vi "PH_BackreflectionMeas.get relevant Data.vi"(0 "i ref in":refnum<vi>, 5 "error in":errorcluster) -> (14 "i ref out":refnum<vi>, 16 "low Energy Waveform":waveform(dbl), 17 "high Energy Waveform":waveform(dbl), 19 "error out":errorcluster)   [LabVIEW 2014, in "PH_BackreflectionMeas.lvlib"]
doc: "This VI gets - depending on the Alignment or shot Mode - the relevant data."
uses:
  PH_BackreflectionMeas.lvlib
  PH_Devices/PH_TKTDS-30xx/PH_TKTDS-30xx.lvlib
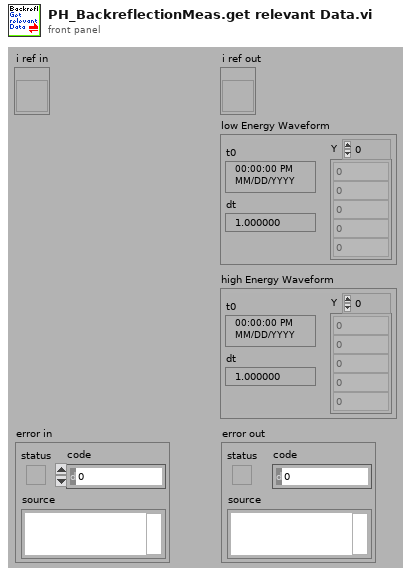
[diagram p1: front panel]
types:
  T1 = typedef "PH_TKTDS-30xx.lvlib/PH_TKTDS-30xx.i attribute.ctl" = cluster{"Default VISA Resource":string, "VISA Resource Name":refnum<visa-resource-name>, "Revision":cluster{"Instrument Driver":string, "Instrument Firmware":string}, "Selftest":cluster{"Result":u32, "Message":string}, "Channels":T2[], "Trigger Configuration":T4, "Acquisition Configuration":T5, "Fetched Waveforms":T6[], "GUI Refs":T7, "State":T8, "Error Message":string, "Allow Prdc Loop?":bool}
  T2 = typedef "PH_TKTDS-30xx.lvlib/PH_TKTDS-30xx.Channel Config.ctl" = cluster{"Channel Name":string, "Input Impedance":string, "Max Input Frequency":string, "Vertical Coupling":i32, "Channel Enabled":bool, "Probe Attenuation":dbl, "Vertical Range":dbl, "Vertical Offset":dbl, "Waveform Limits":T3}
  T3 = typedef "PH_TKTDS-30xx.lvlib/PH_TKTDS-30xx.Waveform Limits.ctl" = cluster{"Start":i32, "End":i32}
  T4 = typedef "PH_TKTDS-30xx.lvlib/PH_TKTDS-30xx.Trigger Config.ctl" = cluster{"Source":string, "Slope":i32, "Level [V]":dbl}
  T5 = typedef "PH_TKTDS-30xx.lvlib/PH_TKTDS-30xx.Acquisition Config.ctl" = cluster{"Time base":dbl, "Record Length":u16, "Start Time":dbl, "Type":i32, "Continuous":bool}
  T6 = typedef "PH_TKTDS-30xx.lvlib/PH_TKTDS-30xx.fetched Waveform.ctl" = cluster{"Source":string, "Actual Points":u32, "Initial X":dbl, "X Increment":dbl, "Waveform Array":dbl[]}
  T7 = typedef "PH_TKTDS-30xx.lvlib/PH_TKTDS-30xx.GUI Refs.ctl" = cluster{"Trigger":refnum<vi>, "Acquisition":refnum<vi>, "State":refnum<vi>, "Delete":refnum<vi>, "Channel to be positioned":refnum<vi>, "Postion":refnum<vi>, "Display Intensity":refnum<vi>, "VISA Resource":refnum<vi>, "Channels":refnum<vi>[], "Graphs":refnum<vi>[]}
  T8 = typedef "PH_StatusHandler.lvlib/PH_StatusHandler.Status.ctl" = i16
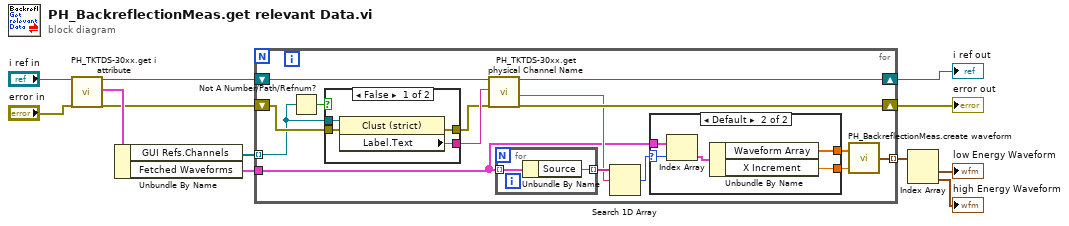
[diagram p0: block diagram]
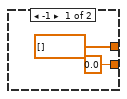
[diagram p2: hidden frame]
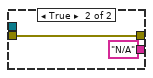
[diagram p3: hidden frame]
diagram:
  n1 = call "PH_TKTDS-30xx.get i attribute.vi"("i ref in"="i ref in", "error in (no error)"="error in") -> ("i ref out"=w7:refnum<vi>, "i attribute"=w12:T1, "error out"=w10:errorcluster)  [unwired: 15 in]
  n2 = Unbundle By Name(w12) -> ("GUI Refs.Channels"=w11:refnum<vi>[], "Fetched Waveforms"=w6:T6[])
  n3 = for {
    shift-right: [w21] -> w1
    shift-left: w10 -> [w27]
    tunnel: w11 -> [w25] mode=indexing
    shift-right: [w22] -> w2
    shift-left: w7 -> [w23]
    tunnel: w6 -> [w16]
    tunnel: [w13] -> w5 mode=indexing
    n4 = Not A Number/Path/Refnum?(number/path/refnum=w25) -> (NaN/Path/Refnum?=w26:bool)
    n5 = case shown="False" w26 {
      tunnel: w27 -> [w40 w42]
      tunnel: [w39 w42] -> w20
      tunnel: [w38 "N/A" ("Label.Text")] -> w24
      tunnel: w25 -> [w37 _]
      frame False {
        n6 = property class="Clust (strict)"(reference=w37, error in=w40) -> (error out=w39:errorcluster, "Label.Text"=w38:string)  [unwired: 1 out]
      }
      frame True {
      }
    }
    n7 = call "PH_TKTDS-30xx.get physical Channel Name.vi"("i ref in"=w23, "GUI Element Name"=w24, "error in"=w20) -> ("i ref out"=w22:refnum<vi>, "Physical Channel Name"=w18:string, "error out"=w21:errorcluster)  [unwired: 13 in, 1 out]
    n8 = for {
      tunnel: w16 -> [w36] mode=indexing
      tunnel: [w35] -> w19 mode=indexing
      n9 = Unbundle By Name(w36) -> ("Source"=w35:string)
    }
    n10 = Search 1D Array(1D array=w19, element=w18) -> (index of element=w17:i32)  [unwired: 1 in]
    n11 = case shown="Default" w17 {
      selector: w17 -> [_ w31]
      tunnel: w16 -> [_ w34]
      tunnel: [0.0 ("X Increment") w30] -> w14
      tunnel: [dbl[] [] ("Waveform Array") w32] -> w15
      frame -1 {
      }
      frame Default {
        n12 = Index Array(array=w34, index=w31) -> (element=w33:T6)
        n13 = Unbundle By Name(w33) -> ("Waveform Array"=w32:dbl[], "X Increment"=w30:dbl)
      }
    }
    n14 = call "PH_BackreflectionMeas.create waveform.vi"("dt"=w14, "Y-Data"=w15) -> ("waveform out"=w13:waveform(dbl))
  }
  "error out" <- w1
  "i ref out" <- w2
  n15 = Index Array(array=w5) -> (element #1=→"low Energy Waveform":waveform(dbl), element #2=→"high Energy Waveform":waveform(dbl))  [unwired: 2 in]
